vi "xml example.vi"() -> ()   [LabVIEW 2012]
uses:
  <vilib>/xml/NI_XML.lvlib
  <resource>/objmgr/DOMUserDefRef.rc
  <vilib>/xml/Close Reference(Node).vi
panel:
  out "Node Name":string
  in  "XML String 4":string="<a attr = \"attr1\"><b>b1</b><b>b2</b></a>"
  in  "XML String 3":string="<a attr = \"attr1\"><b>b1</b><b>b2</b></a>"
  in  "Tree":string(tree)
  in  "XML String 2":string="<a attr = \"attr1\"><b>b1</b><b>b2</b></a>"
  out "error out":errorcluster
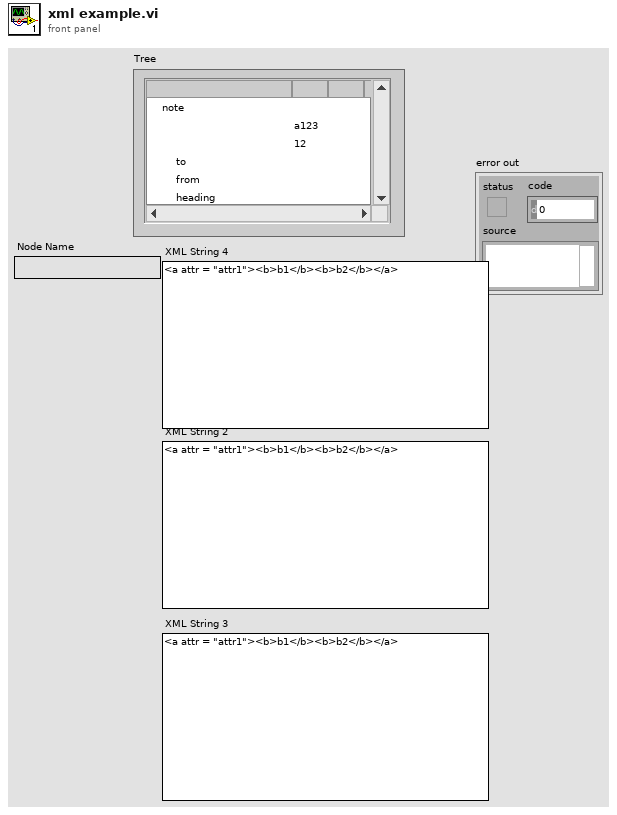
[diagram p1: front panel]
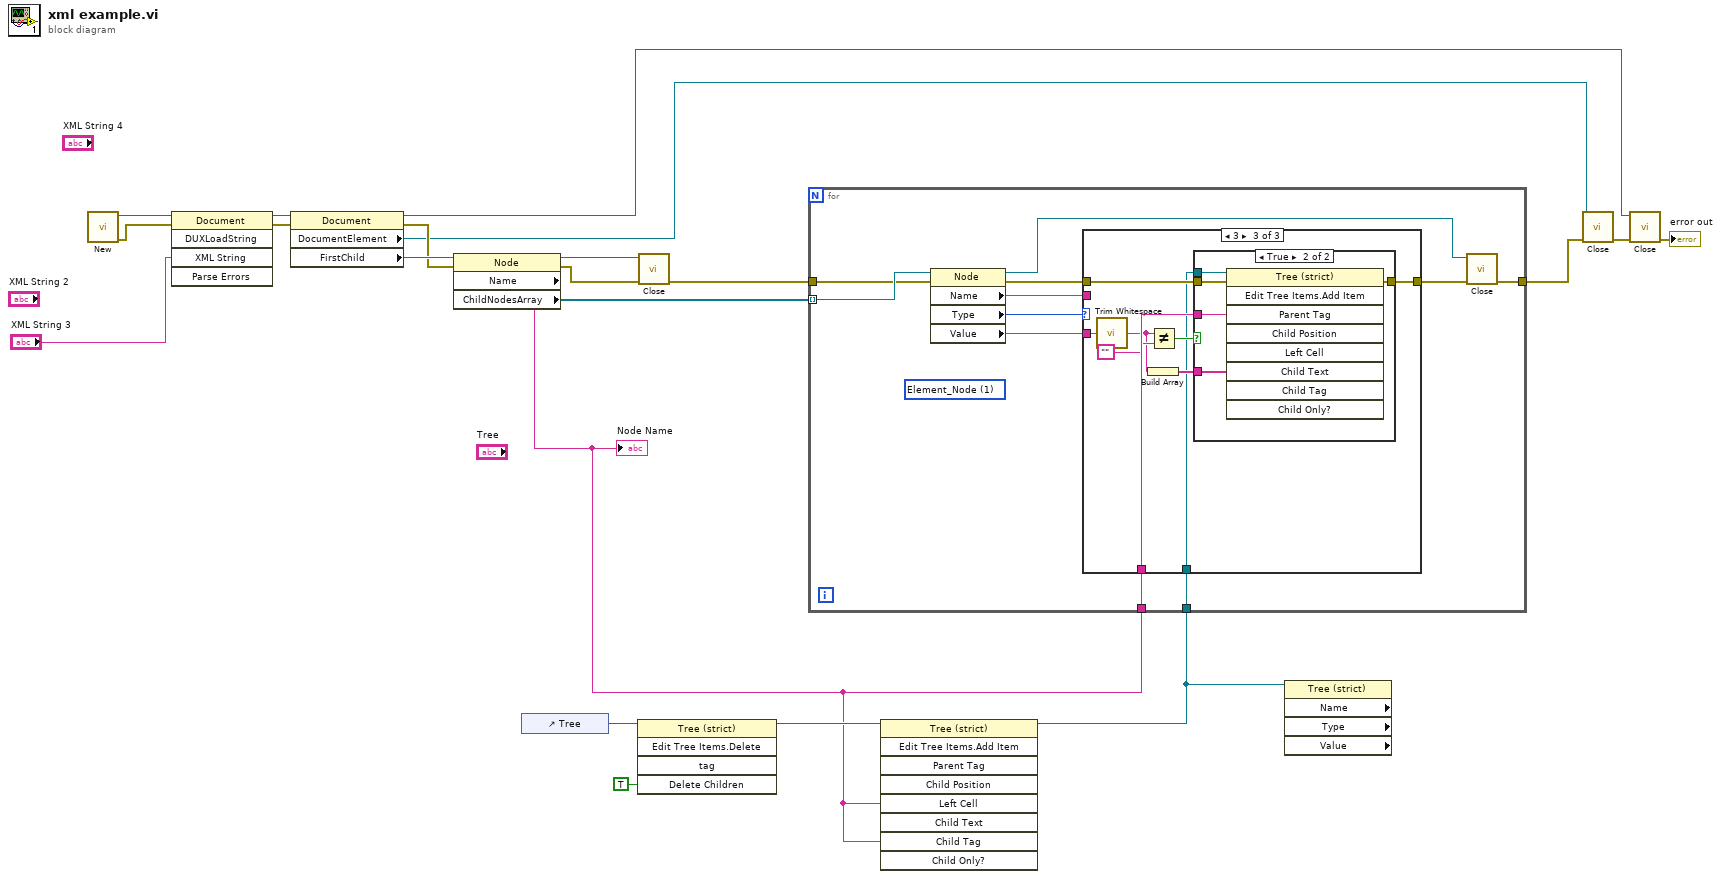
[diagram p0: block diagram]
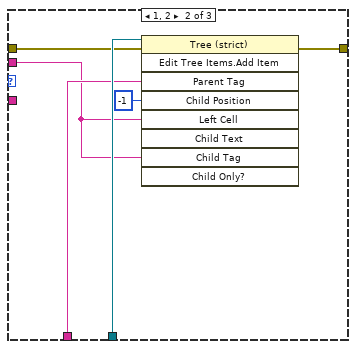
[diagram p3: hidden frame]
diagram:
  n1 = call <vilib>:"New.vi"() -> ("error out"=w20:errorcluster, "DOM document out"=w21:refnum<k20>)  [unwired: 8 in]
  n2 = invoke class="Document" method="DUXLoadString"(reference=w21, error in=w20, "XML String"="XML String 3") -> (reference out=w18:refnum<k20>, error out=w17:errorcluster)  [unwired: 2 in, 3 out]
  n3 = property class="Document"(reference=w18, error in=w17) -> (reference out=w13:refnum<k20>, error out=w10:errorcluster, "DocumentElement"=w3:refnum<k20>, "FirstChild"=w11:refnum<k20>)
  n4 = property class="Node"(reference=w11, error in=w10) -> (reference out=w9:refnum<k20>, error out=w8:errorcluster, "Name"=w7:string, "ChildNodesArray"=w6:refnum<k20>[])
  "Node Name" <- w7
  n5 = control-ref of="Tree"() -> (w16:refnum<vi>)
  n6 = invoke class="Tree (strict)" method="Edit Tree Items.Delete"(reference=w16, "Delete Children"=TRUE ("Delete Children?")) -> (reference out=w15:refnum<vi>)  [unwired: 3 in, 4 out]
  n7 = call-poly <vilib>:"Close.vi"("error in (no error)"=w8, "node"=w9) -> ("error out"=w5:errorcluster)  [unwired: 7 in]
  n8 = invoke class="Tree (strict)" method="Edit Tree Items.Add Item"(reference=w15, "Left Cell"=w7, "Child Tag"=w7) -> (reference out=w1:refnum<vi>)  [unwired: 6 in, 8 out]
  n9 = for {
    tunnel: w6 -> [w25] mode=indexing
    tunnel: w5 -> [w24]
    tunnel: w1 -> [w32]
    tunnel: [w31] -> w4
    tunnel: w7 -> [w30]
    (unwired) 1 items=["Element_Node"=1, "Attribute_Node"=2, "Text_Node"=3, "CDATASection_Node"=4, "EntityReference_Node"=5, "Entity_Node"=6, "ProcessingInstruction_Node"=7, "Comment_Node"=8, "Document_Node"=9, "DocumentType_Node"=10, "DocumentFragment_Node"=11, "Notation_Node"=12] ("Node Type")
    n10 = property class="Node"(reference=w25, error in=w24) -> (reference out=w26:refnum<k20>, error out=w28:errorcluster, "Name"=w27:string, "Type"=w23:i32, "Value"=w22:string)
    n11 = case shown="3" w23 {
      tunnel: w32 -> [_ w39 w40]
      tunnel: w30 -> [_ w37 w46]
      tunnel: [w33 w36 w47] -> w29
      tunnel: w28 -> [w33 w35 w48]
      tunnel: w27 -> [_ w34 _]
      tunnel: w22 -> [_ _ w45]
      frame 0, Default {
      }
      frame 1, 2 {
        n12 = invoke class="Tree (strict)" method="Edit Tree Items.Add Item"(reference=w39, error in=w35, "Parent Tag"=w37, "Child Position"=-1, "Left Cell"=w34, "Child Tag"=w34) -> (error out=w36:errorcluster)  [unwired: 3 in, 8 out]
      }
      frame 3 {
        n13 = call <vilib>:"Trim Whitespace.vi"("string"=w45) -> ("trimmed string"=w41:string)  [unwired: 1 in]
        n14 = Build Array(w41) -> (w42:string[])
        n15 = Not Equal?(x=w41, y="") -> (x != y?=w43:bool)
        n16 = case shown="True" w43 {
          tunnel: w48 -> [w49 w54]
          tunnel: [w49 w53] -> w47
          tunnel: w46 -> [_ w52]
          tunnel: w42 -> [_ w51]
          tunnel: w40 -> [_ w50]
          frame False {
          }
          frame True {
            n17 = invoke class="Tree (strict)" method="Edit Tree Items.Add Item"(reference=w50, error in=w54, "Parent Tag"=w52, "Child Text"=w51) -> (error out=w53:errorcluster)  [unwired: 5 in, 8 out]
          }
        }
      }
    }
    n18 = call-poly <vilib>:"Close.vi"("error in (no error)"=w29, "node"=w26) -> ("error out"=w31:errorcluster)  [unwired: 7 in]
  }
  n19 = property class="Tree (strict)" props=["Name", "Type", "Value"](reference=w1) -> ()  [unwired: 1 in, 5 out]
  n20 = call-poly <vilib>:"Close.vi"("error in (no error)"=w4, "node"=w3) -> ("error out"=w12:errorcluster)  [unwired: 7 in]
  n21 = call-poly <vilib>:"Close.vi"("error in (no error)"=w12, "node"=w13) -> ("error out"=→"error out":errorcluster)  [unwired: 7 in]
